vi "Build All.vi"() -> ()   [LabVIEW 2015]
uses:
  <vilib>/AppBuilder/AB_API_Simple/Build (path).vi
  <vilib>/AppBuilder/AB_API_Simple/NI_App_Builder_API.lvlib
panel:
  in  "String":string
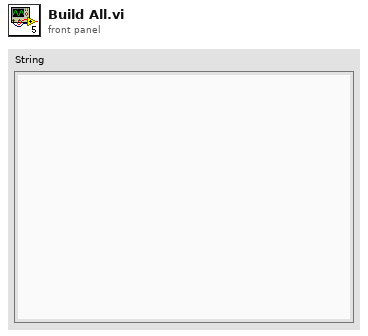
[diagram p1: front panel]
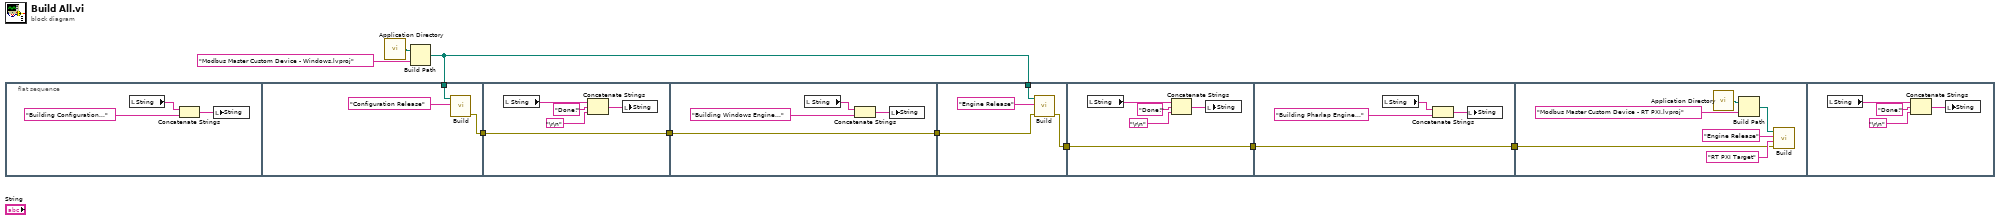
[diagram p0: block diagram]
diagram:
  n1 = flat-sequence {
    tunnel: w7 -> [w14]
    tunnel: [w13] -> w4
    tunnel: [w16] -> w5
    tunnel: w4 -> [w16]
    tunnel: [w21] -> w6
    tunnel: w5 -> [w21]
    tunnel: w7 -> [w27]
    tunnel: w6 -> [w26]
    tunnel: [w25] -> w1
    tunnel: [w29] -> w2
    tunnel: w1 -> [w29]
    tunnel: [w34] -> w3
    tunnel: w2 -> [w34]
    tunnel: w3 -> [w38]
    frame #0 {
      n2 = local read "String"() -> (w10:string)
      n3 = Concatenate Strings(w10, "Building Configuration..." ("String")) -> (w12:string)
      n4 = local write "String"(w12) -> ()
    }
    frame #1 {
      n5 = call-poly <vilib>:"Build.vi"("Name of build specification (if empty: build all)"="Configuration Release", "Path to project"=w14) -> ("error out"=w13:errorcluster)  [unwired: 8 in, 1 out]
    }
    frame #2 {
      n6 = local read "String"() -> (w20:string)
      n7 = Concatenate Strings(w20, "Done!" ("String"), "\r\n") -> (w18:string)
      n8 = local write "String"(w18) -> ()
    }
    frame #3 {
      n9 = local read "String"() -> (w24:string)
      n10 = Concatenate Strings(w24, "Building Windows Engine..." ("String")) -> (w22:string)
      n11 = local write "String"(w22) -> ()
    }
    frame #4 {
      n12 = call-poly <vilib>:"Build.vi"("error in (no error)"=w26, "Name of build specification (if empty: build all)"="Engine Release", "Path to project"=w27) -> ("error out"=w25:errorcluster)  [unwired: 7 in, 1 out]
    }
    frame #5 {
      n13 = local read "String"() -> (w30:string)
      n14 = Concatenate Strings(w30, "Done!" ("String"), "\r\n") -> (w32:string)
      n15 = local write "String"(w32) -> ()
    }
    frame #6 {
      n16 = local read "String"() -> (w35:string)
      n17 = Concatenate Strings(w35, "Building Pharlap Engine..." ("String")) -> (w37:string)
      n18 = local write "String"(w37) -> ()
    }
    frame #7 {
      n19 = call <vilib>:"Application Directory.vi"() -> ("Application Directory"=w39:path)
      n20 = Build Path(base path=w39, name or relative path="Modbus Master Custom Device - RT PXI.lvproj") -> (appended path=w40:path)
      n21 = call-poly <vilib>:"Build.vi"("error in (no error)"=w38, "Name of target (My Computer)"="RT PXI Target", "Name of build specification (if empty: build all)"="Engine Release", "Path to project"=w40) -> ()  [unwired: 6 in, 2 out]
    }
    frame #8 {
      n22 = local read "String"() -> (w47:string)
      n23 = Concatenate Strings(w47, "Done!" ("String"), "\r\n") -> (w45:string)
      n24 = local write "String"(w45) -> ()
    }
  }
  n25 = call <vilib>:"Application Directory.vi"() -> ("Application Directory"=w9:path)
  n26 = Build Path(base path=w9, name or relative path="Modbus Master Custom Device - Windows.lvproj") -> (appended path=w7:path)
